vi "Send Message.vi"(5 "Target Task":string, 7 "Target ID":u32, 8 "error in (no error)":errorcluster, 9 "Type":string, 10 "Payload":u8[](array[numeric]), 11 "TCPMessageService in":refnum<class "TCPMessageAPI.lvclass">) -> (0 "error out":errorcluster, 3 "TCPMessageService out":refnum<class "TCPMessageAPI.lvclass">)   [LabVIEW 2020, in "Vecto.lvlib" / "TCPMessageAPI.lvclass"]
uses:
  TCPMessageAPI.lvclass
  Send Message Data.ctl
  lv-volatus/messages/TcpPayload/Data.ctl
  lv-promises/Promises/Promise/Promise.lvclass
  TCPMessageAPI.lvclass/TCPMessageAPI.ctl
  lv-volatus/messages/TcpPayload/TcpPayload.lvlib
  Vecto.lvlib
  TCPMessaging/TCPMessaging.lvclass
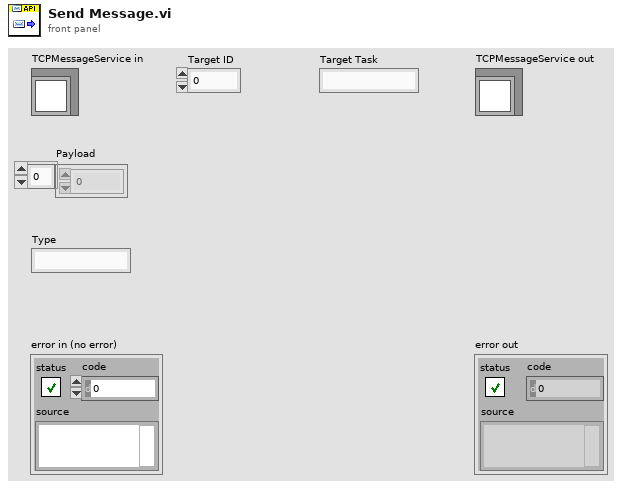
[diagram p1: front panel]
types:
  T1 = typedef "Vecto.lvlib/Send Message Data.ctl" = cluster{"TcpPayload":T2, "Register Reply":bool, "Reply Promise":refnum<class "Promise.lvclass">, "Reply Deadline":dbl}
  T2 = typedef "TcpPayload.lvlib/Data.ctl" = cluster{"target_node":u32, "source_id":u32, "sequence":u32, "timestamp":i64, "type":string, "task_id":string, "payload":u8[]}
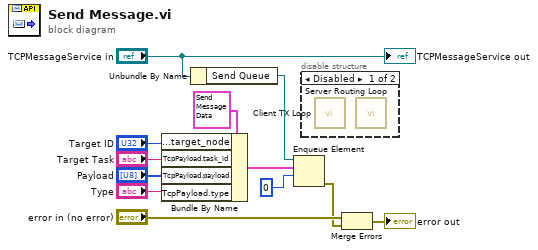
[diagram p0: block diagram]
diagram:
  n1 = Bundle By Name(cluster=T1 {"TcpPayload"={"target_node"=0, "source_id"=0, "sequence"=0, "timestamp"=0, "type"="", "task_id"="", "payload"=[]}, "Register Reply"=FALSE, "Reply Promise"=refnum, "Reply Deadline"=0.0} ("Send Message Data"), "TcpPayload.target_node"="Target ID", "TcpPayload.task_id"="Target Task", "TcpPayload.payload"="Payload", "TcpPayload.type"="Type") -> (w1:T1)
  n2 = Unbundle By Name("TCPMessageService in") -> ("Send Queue"=w6:refnum<queue>)
  n3 = Enqueue Element(queue=w6, element=w1, timeout in ms (-1)=0) -> (error out=w2:errorcluster)  [unwired: 1 in, 2 out]
  n4 = disable-structure shown="Disabled" {
    frame Disabled {
      n5 = call "Client TX Loop.vi"() -> ()  [unwired: 11 in, 1 out]
      n6 = call "Server Routing Loop.vi"() -> ()  [unwired: 11 in, 1 out]
    }
    frame Enabled {
    }
  }
  n7 = Merge Errors("error in (no error)", w2) -> (→"error out":errorcluster)
  "TCPMessageService out" <- "TCPMessageService in"
